vi "SendRef.vi"(8 "error in (no error)":errorcluster, 11 "Instrument in":refnum<class "Instrument.lvclass">) -> (0 "error out":errorcluster, 3 "Instrument out":refnum<class "Instrument.lvclass">)   [LabVIEW 2018, in "Instrument.lvclass"]
uses:
  Instrument.lvclass
  C:/Users/observer/Desktop/Sparc4GUI/SPARC4_GUI/Server/Server.lvclass
  Server/Server.lvclass/Server.ctl
  Server/Server.lvclass
panel:
  out "output cluster":cluster{"Address":string, "Remote Port":u32}
  in  "Cluster":cluster{"Address":string, "Remote Port":u32}
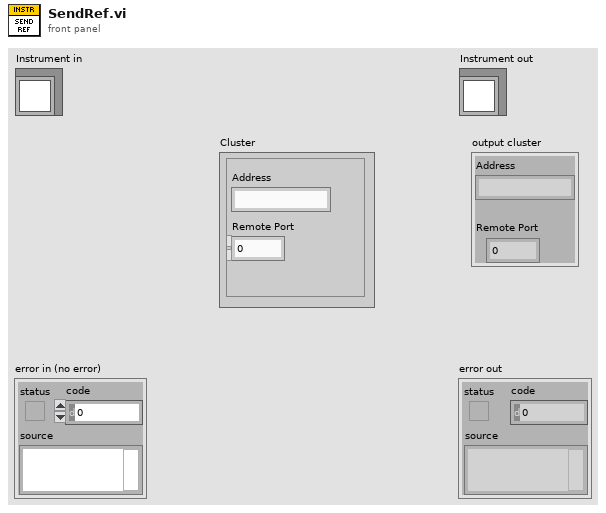
[diagram p1: front panel]
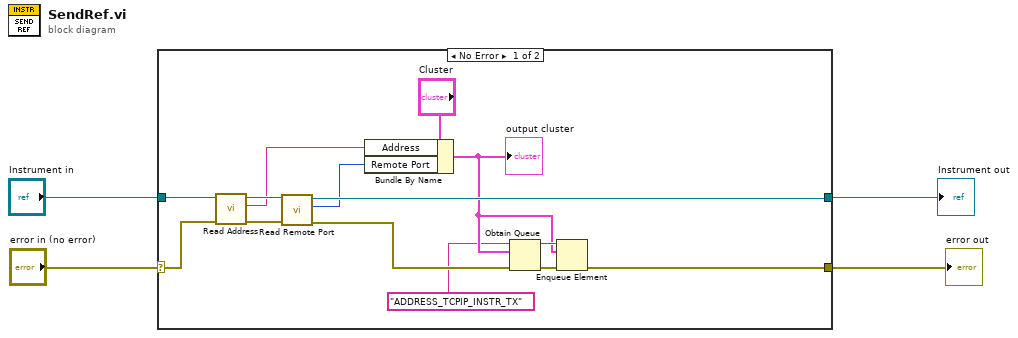
[diagram p0: block diagram]
diagram:
  n1 = case shown="No Error" "error in (no error)" {
    selector: "error in (no error)" -> [w14 w20]
    tunnel: [w5 w20] -> w1
    tunnel: [w12 w19] -> w2
    tunnel: "Instrument in" -> [w15 w19]
    frame No Error {
      n2 = call "Read Address.vi"("error in (no error)"=w14, "Server in"=w15) -> ("error out"=w8:errorcluster, "Address"=w11:string, "Server out"=w13:refnum<class "Instrument.lvclass">)  [unwired: 7 in]
      n3 = call "Read Remote Port.vi"("error in (no error)"=w8, "Server in"=w13) -> ("error out"=w7:errorcluster, "Remote Port"=w10:u32, "Server out"=w12:refnum<class "Instrument.lvclass">)  [unwired: 7 in]
      n4 = Bundle By Name(cluster="Cluster", "Address"=w11, "Remote Port"=w10) -> (w9:cluster{"Address":string, "Remote Port":u32})
      "output cluster" <- w9
      n5 = Obtain Queue(name (unnamed)="ADDRESS_TCPIP_INSTR_TX", element data type=w9, error in (no error)=w7) -> (queue out=w18:refnum<queue>, error out=w17:errorcluster)  [unwired: 2 in, 1 out]
      n6 = Enqueue Element(queue=w18, element=w9, error in (no error)=w17) -> (error out=w5:errorcluster)  [unwired: 1 in, 2 out]
    }
    frame Error {
    }
  }
  "error out" <- w1
  "Instrument out" <- w2
